vi "Main.vi"(8 "error in":errorcluster, 11 "Graph Master in":refnum<class "Graph Master.lvclass">) -> (0 "error out":errorcluster, 3 "Graph Master out":refnum<class "Graph Master.lvclass">)   [LabVIEW 2023, in "Graph Master.lvclass"]
doc: "The <b>Queued Message Handler</b> of the Worker that owns this VI."
uses:
  Graph Master.lvclass
  C:/Program Files/National Instruments/LabVIEW 2023/vi.lib/addons/_Workers/Library/Classes/Worker/Worker.lvclass
  Initialization Data.ctl
  Response Cases.ctl
  Graph Master.lvclass/Graph Master.ctl
  rqp_Create Graph.ctl
  GraphUI/Initialization Data.ctl
  GraphUI/Response Cases.ctl
  GraphUI/GraphUI.lvclass
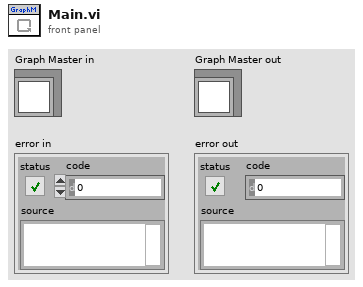
[diagram p1: front panel]
types:
  T1 = typedef "Graph Master.lvclass/Initialization Data.ctl" = cluster{"Response Cases":T2}
  T2 = typedef "Graph Master.lvclass/Response Cases.ctl" = cluster{"Placeholder - Can be deleted":string}
  T3 = typedef "GraphUI.lvclass/Initialization Data.ctl" = cluster{"Response Cases":T4, "Control ref":refnum<vi>}
  T4 = typedef "GraphUI.lvclass/Response Cases.ctl" = cluster{"Placeholder - Can be deleted":string}
  T5 = typedef "Graph Master.lvclass/rqp_Create Graph.ctl" = cluster{"Control ref":refnum<vi>}
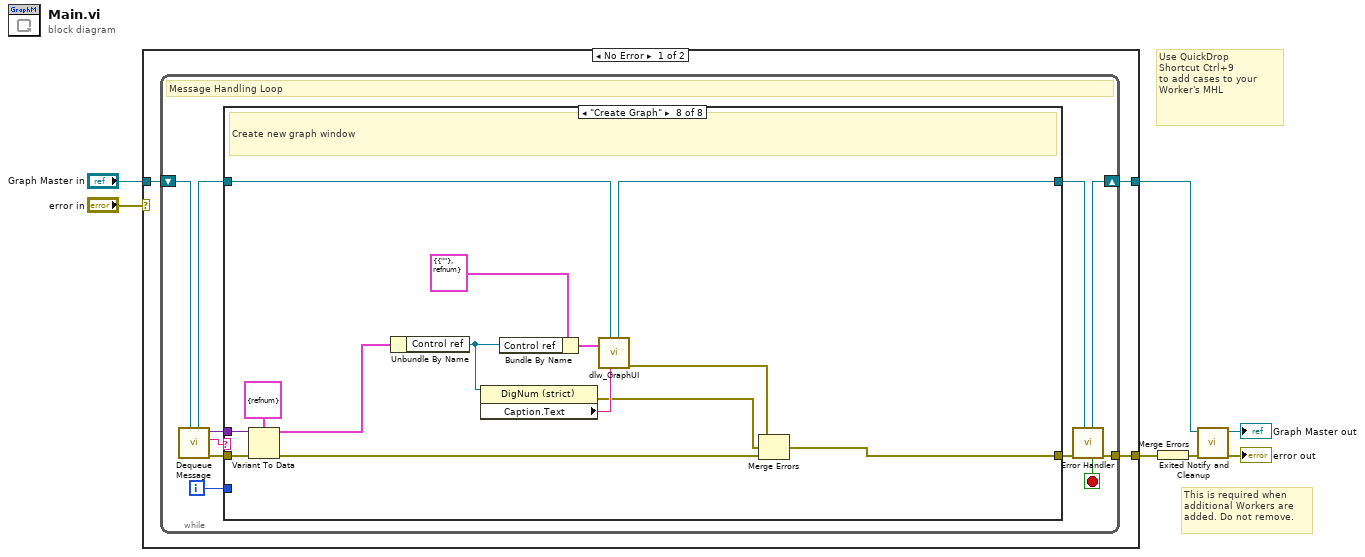
[diagram p0: block diagram]
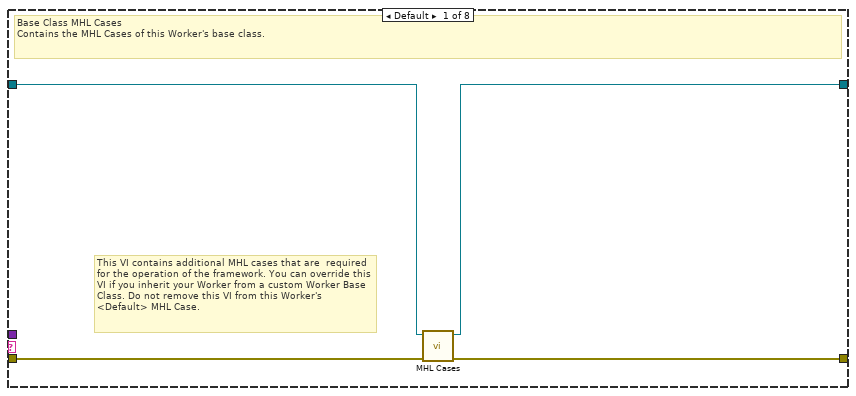
[diagram p2: hidden frame]
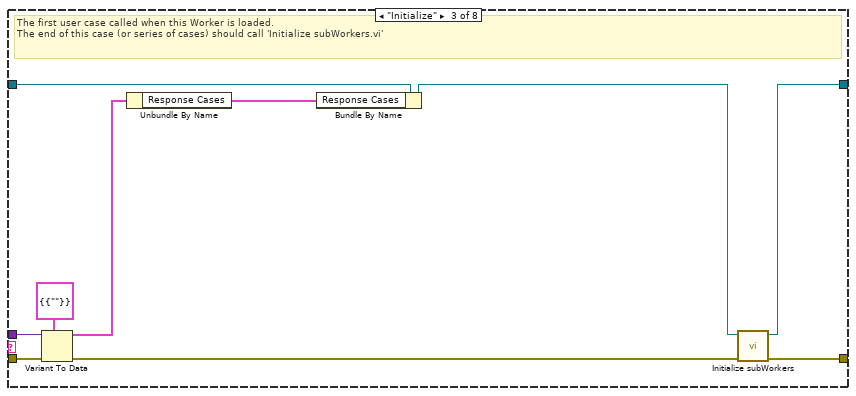
[diagram p4: hidden frame]
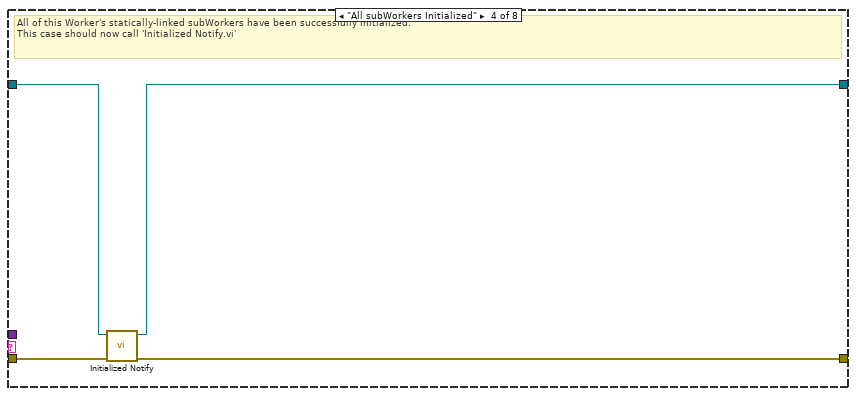
[diagram p5: hidden frame]
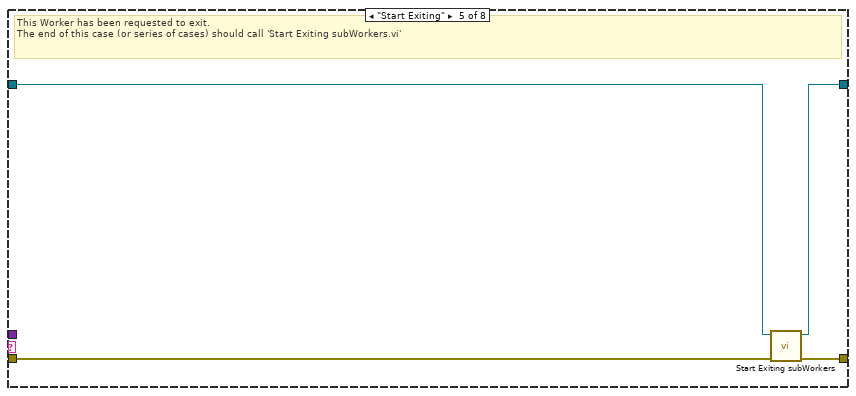
[diagram p6: hidden frame]
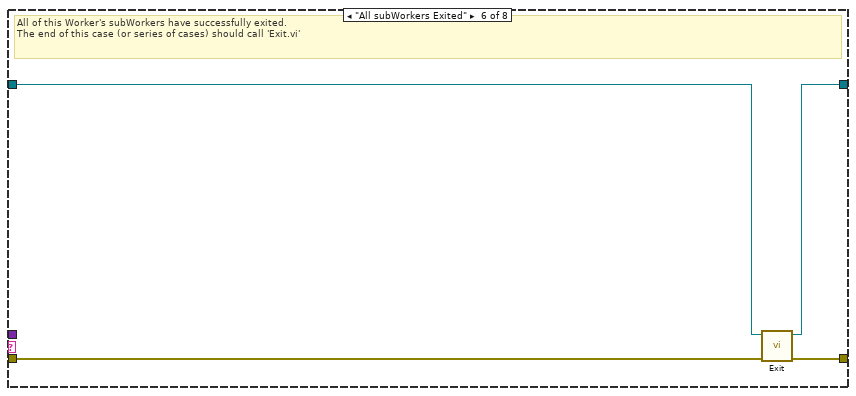
[diagram p7: hidden frame]
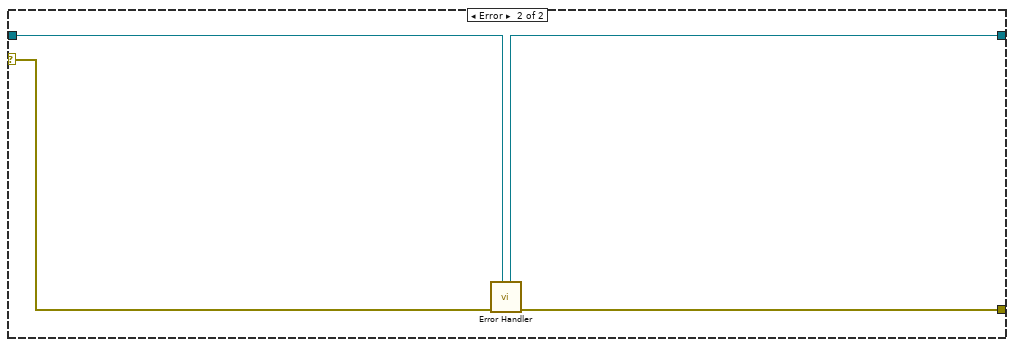
[diagram p9: hidden frame]
diagram:
  # "Use QuickDrop\nShortcut Ctrl+9\nto add cases to your\nWorker's MHL"
  # "This is required when additional Workers are added. Do not remove."
  n1 = case shown="No Error" "error in" {
    tunnel: "Graph Master in" -> [w8 w67]
    tunnel: [w10 w68] -> w6
    tunnel: [w9 w66] -> w7
    selector: "error in" -> [_ w69]
    frame No Error {
      n2 = while {
        shift-right: [w19] -> w9
        shift-left: w8 -> [w21]
        tunnel: [w20] -> w10
        i -> [w12]
        stop <- w13 stop-if-true
        # "Message Handling Loop"
        n3 = call-dynamic "Dequeue Message.vi"("Worker"=w21) -> ("error out"=w18:errorcluster, "Case out"=w14:string, "Data out"=w11:variant, "Worker out"=w16:refnum<class "Graph Master.lvclass">)  [unwired: 6 in, 1 out]
        n4 = case "Worker MHL Case Structure (DO NOT CHANGE LABEL NAME)" shown="\"Create Graph\"" w14 {
          tunnel: w18 -> [w25 w26 w35 w41 w42 w49 w51 w65]
          tunnel: [w24 w26 w37 w40 w45 w48 w51 w60] -> w17
          tunnel: w16 -> [w23 w27 w34 w39 w43 w47 w50 w59]
          tunnel: [w22 w27 w36 w38 w44 w46 w50 w58] -> w15
          tunnel: w12 -> [_ _ _ _ _ _ _ _]
          tunnel: w11 -> [_ _ w32 _ _ _ _ w62]
          frame Default {
            # "This VI contains additional MHL cases that are  required for the operation of the framework. You can override this VI if you inherit your Worker from a custom Worker Base Class. Do not remove this VI from this Worker's <Default> MHL Case."
            # "Base Class MHL Cases\nContains the MHL Cases of this Worker's base class."
            n5 = call-dynamic "MHL Cases.vi"("error in"=w25, "Worker in"=w23) -> ("error out"=w24:errorcluster, "Worker out"=w22:refnum<class "Graph Master.lvclass">)  [unwired: 8 in]
          }
          frame "------------ FRAMEWORK CASES -----------" {
            # "Start of Workers Framework Cases"
          }
          frame "Initialize" {
            # "The first user case called when this Worker is loaded.\nThe end of this case (or series of cases) should call 'Initialize subWorkers.vi'"
            n6 = Variant To Data(error in=w35, type=T1 {"Response Cases"={"Placeholder - Can be deleted"=""}} ("Cluster"), Variant=w32) -> (data=w30:T1, error out=w33:errorcluster)
            n7 = Unbundle By Name(w30) -> ("Response Cases"=w29:T2)
            n8 = Bundle By Name(cluster=w34, "Response Cases"=w29) -> (w31:refnum<class "Graph Master.lvclass">)
            n9 = call-dynamic "Initialize subWorkers.vi"("error in"=w33, "Worker"=w31) -> ("error out"=w37:errorcluster, "dup Worker out"=w36:refnum<class "Graph Master.lvclass">)  [unwired: 8 in]
          }
          frame "All subWorkers Initialized" {
            # "All of this Worker's statically-linked subWorkers have been successfully initialized.\nThis case should now call 'Initialized Notify.vi'"
            n10 = call-dynamic "Initialized Notify.vi"("error in"=w41, "Worker"=w39) -> ("error out"=w40:errorcluster, "dup Worker out"=w38:refnum<class "Graph Master.lvclass">)  [unwired: 8 in]
          }
          frame "Start Exiting" {
            # "This Worker has been requested to exit. \nThe end of this case (or series of cases) should call 'Start Exiting subWorkers.vi'"
            n11 = call-dynamic "Start Exiting subWorkers.vi"("error_in"=w42, "Worker"=w43) -> ("error out"=w45:errorcluster, "dup Worker out"=w44:refnum<class "Graph Master.lvclass">)  [unwired: 8 in]
          }
          frame "All subWorkers Exited" {
            # "All of this Worker's subWorkers have successfully exited. \nThe end of this case (or series of cases) should call 'Exit.vi'"
            n12 = call-dynamic "Exit.vi"("error_in"=w49, "Worker"=w47) -> ("error out"=w48:errorcluster, "dup Worker out"=w46:refnum<class "Graph Master.lvclass">)  [unwired: 8 in]
          }
          frame "------------- PUBLIC API CASES -------------" {
            # "Start of Workers Public API Cases"
          }
          frame "Create Graph" {
            # "Create new graph window"
            n13 = Variant To Data(error in=w65, type=T5 {"Control ref"=refnum} ("Data"), Variant=w62) -> (data=w61:T5, error out=w64:errorcluster)
            n14 = Unbundle By Name(w61) -> ("Control ref"=w55:refnum<vi>)
            n15 = property class="DigNum (strict)"(reference=w55) -> (error out=w53:errorcluster, "Caption.Text"=w54:string)  [unwired: 1 in, 1 out]
            n16 = Bundle By Name(cluster=T3 {"Response Cases"={"Placeholder - Can be deleted"=""}, "Control ref"=refnum} ("Initialization Data"), "Control ref"=w55) -> (w56:T3)
            n17 = call "dlw_GraphUI.vi"("Worker Alias"=w54, "Caller in"=w59, "Initialization Data"=w56) -> ("error out"=w52:errorcluster, "dup Caller out"=w58:refnum<class "Graph Master.lvclass">)  [unwired: 6 in, 1 out]
            n18 = Merge Errors(w52, w53, w64) -> (w60:errorcluster)
          }
        }
        n19 = call-dynamic "Error Handler.vi"("Worker"=w15, "error_in"=w17) -> ("error out"=w20:errorcluster, "Stop Loop"=w13:bool, "Worker out"=w19:refnum<class "Graph Master.lvclass">)  [unwired: 7 in]
      }
    }
    frame Error {
      n20 = call-dynamic "Error Handler.vi"("Worker"=w67, "error_in"=w69) -> ("error out"=w68:errorcluster, "Worker out"=w66:refnum<class "Graph Master.lvclass">)  [unwired: 7 in, 1 out]
    }
  }
  n21 = Merge Errors(w6) -> (w3:errorcluster)
  n22 = call-dynamic "Exited Notify and Cleanup.vi"("error_in"=w3, "Worker"=w7) -> ("error out"=→"error out":errorcluster, "dup Worker out"=→"Graph Master out":refnum<class "Graph Master.lvclass">)  [unwired: 8 in]
